vi "Start.vi"(8 "error in":errorcluster, 11 "Execution Unit Implementation in":refnum<class "Execution Unit.lvclass">) -> (0 "error out":errorcluster, 3 "Execution Unit Implementation out":refnum<class "Execution Unit.lvclass">)   [LabVIEW 2024, in "AIM ARINC 429 Engine.lvlib" / "Implementation.lvlib" / "Execution Unit.lvclass"]
uses:
  Execution Unit.lvclass
  Execution Unit.lvclass/Execution Unit.ctl
  Hardware API/AIM ARINC 429 Hardware API.lvlib
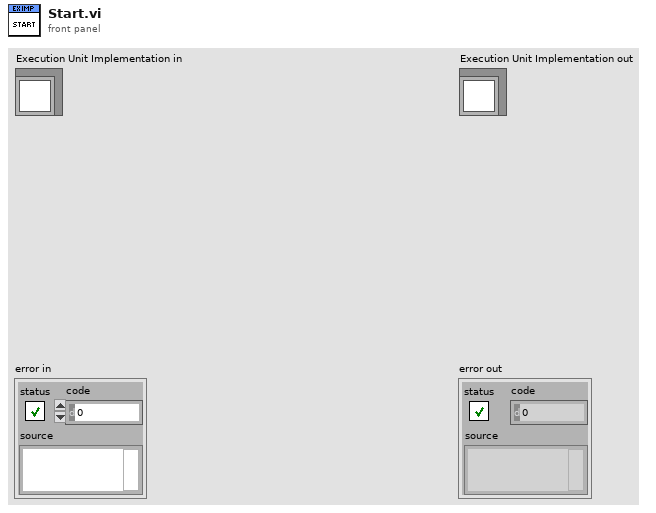
[diagram p1: front panel]
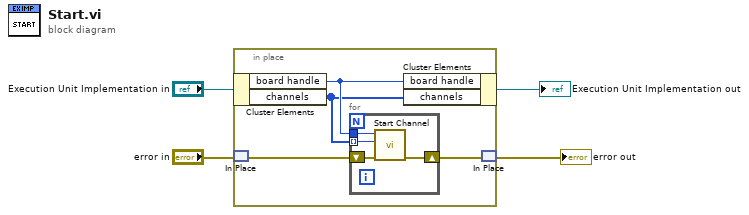
[diagram p0: block diagram]
diagram:
  n1 = in-place {
    n2 = in-place-cluster #1("Execution Unit Implementation in") -> ("board handle"=w7:u8, "channels"=w5:u8[])
    n3 = in-place-match #2("error in") -> (w8:errorcluster)
    n4 = for {
      tunnel: w7 -> [w11]
      shift-right: [w10] -> w6
      shift-left: w8 -> [w12]
      tunnel: w5 -> [w9] mode=indexing
      n5 = call "Start Channel.vi"("error in"=w12, "channel number"=w9, "board handle"=w11) -> ("error out"=w10:errorcluster)  [unwired: 6 in, 2 out]
    }
    n6 = in-place-cluster #1("board handle"=w7, "channels"=w5) -> (→"Execution Unit Implementation out":refnum<class "Execution Unit.lvclass">)
    n7 = in-place-match #2(w6) -> (→"error out":errorcluster)
  }
